vi "保存表格列首设定 (2).vi"(1 "相机光源选项":i32, 2 "ModelEditInfo":T1={"Root"=path "", "AllModelFold"=path "", "AllModelNamePath"=path "", "所有零件型号"=[], "当前零件型号"="", "所有建立零件信息"=[], "当前零件序号"=0, "当前量测零件信息"={"当前点位信息路径"=path "", "量测程式路径"=path "", "当前产品所有量测项目"=[], "当前量测项目序号"=0, "量测项目路径"=path "", "当前产品所有量测项目规格"=[], "参与CPK计算量测项目规格"=[]}, "产品信息"={"产品型号"="J016-9STWH-A插头", "X方向产品数"=1, "X方向间距(mm)"=60.0, "3D相机设定程式序号"=0.0, "扫描行程(mm)"=108.0, "产品检测宽度(默认32mm)"=32.0, "自动抛料?"=FALSE, "校验后才能执行?"=FALSE}} {"当前量测零件信息"."参与CPK计算量测项目规格"."上限" format="%#.4g"; "当前量测零件信息"."参与CPK计算量测项目规格"."下限" format="%#.4g"; "当前量测零件信息"."当前产品所有量测项目规格"."上限" format="%#.4g"; "当前量测零件信息"."当前产品所有量测项目规格"."下限" format="%#.4g"}) -> (0 "表格列首":string[](array[string]))   [LabVIEW 2014]
uses:
  ModelEditSubVIs/ModeEditeControl.ctl
  Controls/TestThreshold.ctl
  ModelEditSubVIs/ModelInfo.ctl
panel:
  # "(1~64)"
  # "~"
  # "~"
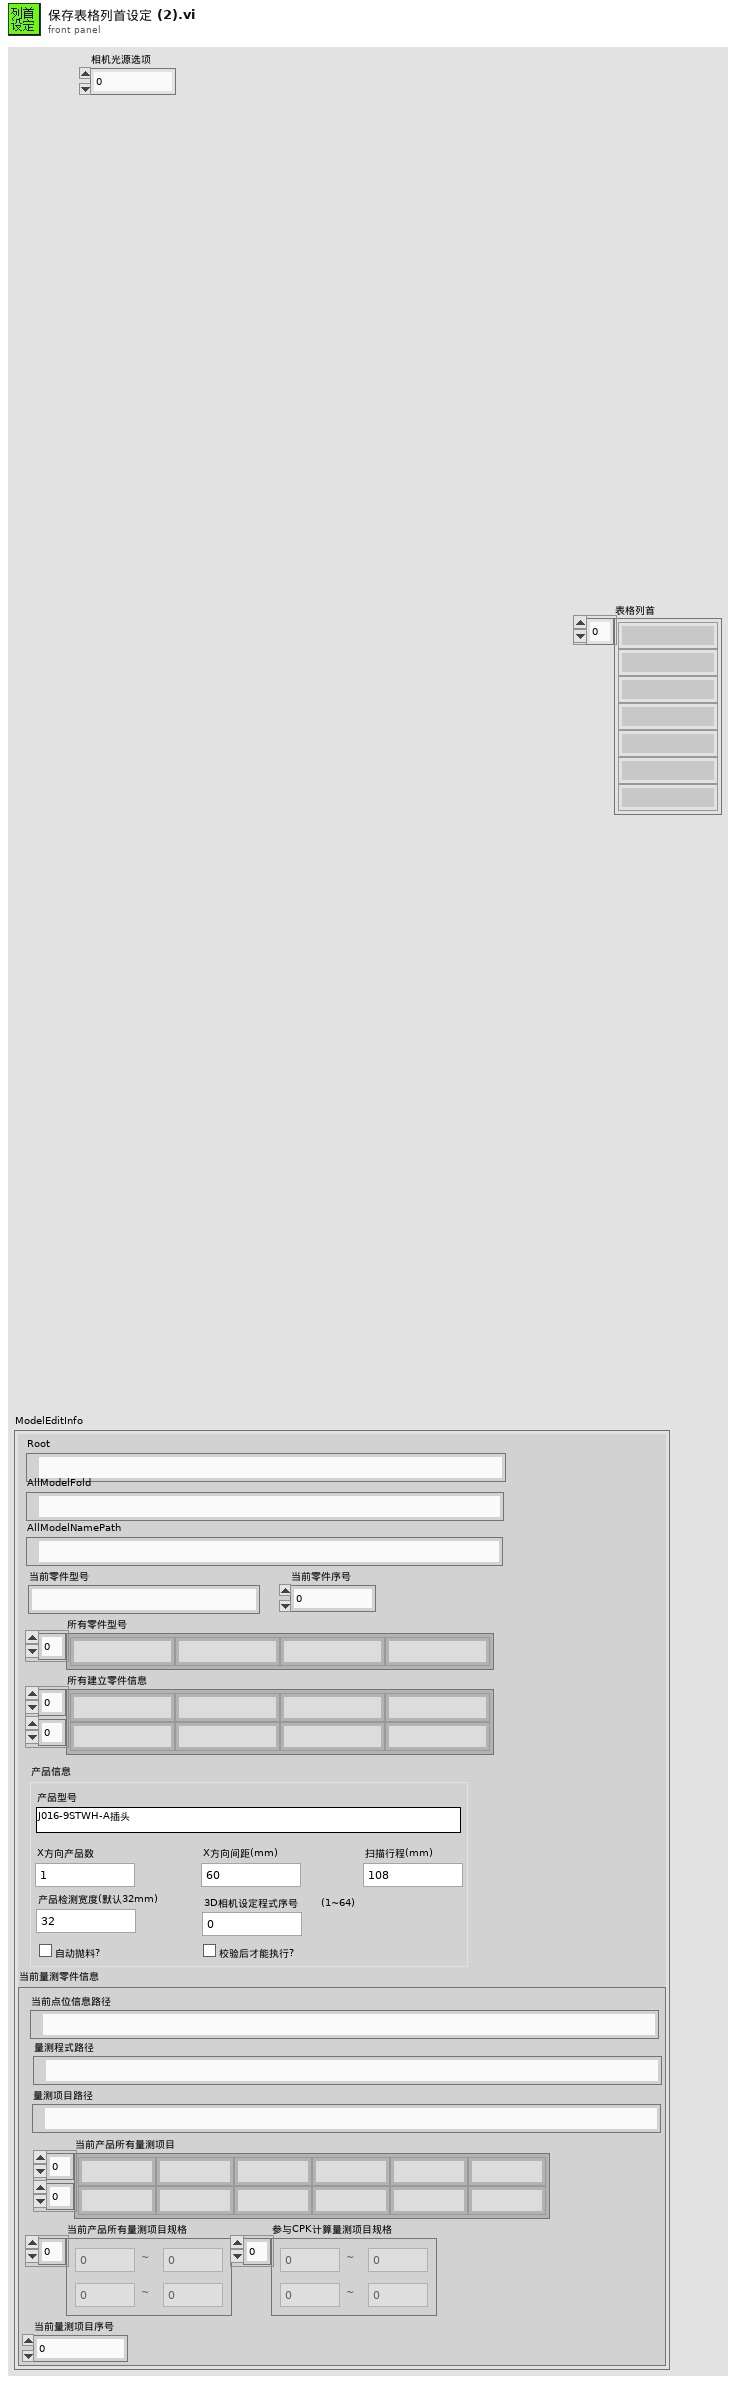
[diagram p1: front panel]
types:
  T1 = typedef "ModeEditeControl.ctl" = cluster{"Root":path, "AllModelFold":path, "AllModelNamePath":path, "所有零件型号":string[], "当前零件型号":string, "所有建立零件信息":string[][], "当前零件序号":i32, "当前量测零件信息":cluster{"当前点位信息路径":path, "量测程式路径":path, "当前产品所有量测项目":string[][], "当前量测项目序号":i32, "量测项目路径":path, "当前产品所有量测项目规格":T2[], "参与CPK计算量测项目规格":T2[]}, "产品信息":T3}
  T2 = typedef "TestThreshold.ctl" = cluster{"下限":dbl, "上限":dbl}
  T3 = typedef "ModelInfo.ctl" = cluster{"产品型号":string, "X方向产品数":i32, "X方向间距(mm)":dbl, "3D相机设定程式序号":dbl, "扫描行程(mm)":dbl, "产品检测宽度(默认32mm)":dbl, "自动抛料?":bool, "校验后才能执行?":bool}
  T4 = typedef "TestItem.ctl" = cluster{"量测项阈值":T2, "量测项目名称":string, "修正系数k":dbl, "单项测试数据个数":i32, "单位mm":bool, "补偿值b":dbl, "下限进位范围":dbl, "上限舍位范围":dbl, "取消测试":bool, "参与CPK计算量测项阈值":T2}
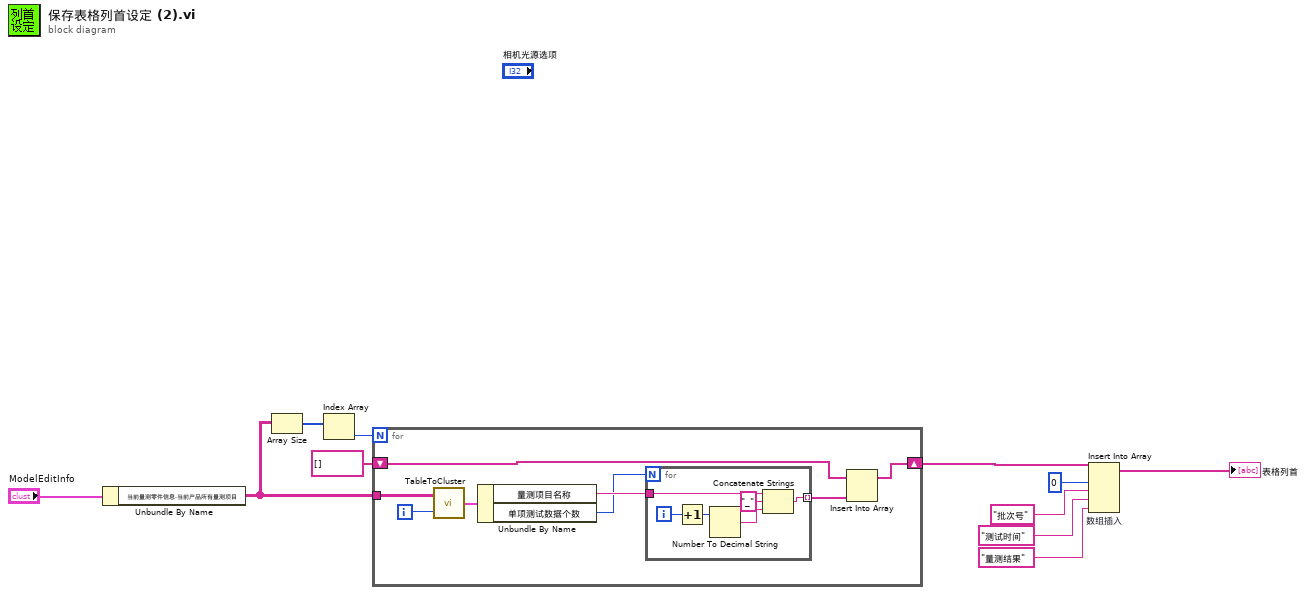
[diagram p0: block diagram]
diagram:
  n1 = Unbundle By Name("ModelEditInfo") -> ("当前量测零件信息.当前产品所有量测项目"=w5:string[][])
  n2 = Array Size(array=w5) -> (size(s)=w4:i32[])
  n3 = Index Array(array=w4) -> (element=w3:i32)  [unwired: 1 in]
  n4 = for {
    N: w3 -> [_]
    tunnel: w5 -> [w19]
    shift-right: [w14] -> w1
    shift-left: string[] [] -> [w13]
    i -> [w18]
    n5 = call "TableToCluster.vi"("Row"=w18, "量测内容"=w19) -> ("量测内容 2"=w17:T4)
    n6 = Unbundle By Name(w17) -> ("量测项目名称"=w16:string, "单项测试数据个数"=w15:i32)
    n7 = for {
      N: w15 -> [_]
      tunnel: w16 -> [w25]
      tunnel: [w22] -> w12 mode=indexing
      i -> [w24]
      n8 = Increment(x=w24) -> (x+1=w23:i32)
      n9 = Number To Decimal String(number=w23) -> (decimal integer string=w21:string)  [unwired: 1 in]
      n10 = Concatenate Strings(w25, "_" ("字符串"), w21) -> (w22:string)
    }
    n11 = Insert Into Array(array=w13, new element=w12) -> (w14:string[])  [unwired: 1 in]
  }
  n12 = Insert Into Array "数组插入"(array=w1, index=0 ("索引"), new element #1="批次号" ("新元素/子数组"), new element #2="测试时间" ("新元素/子数组"), new element #3="量测结果" ("新元素/子数组")) -> (→"表格列首":string[])
